vi "subvi2.vi"(10 "Numeric in":i32, 11 "Motor Step/Direction":u16) -> (3 "Numeric out":u32)   [LabVIEW 2018]
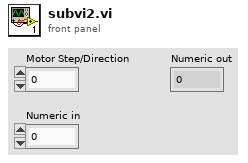
[diagram p1: front panel]
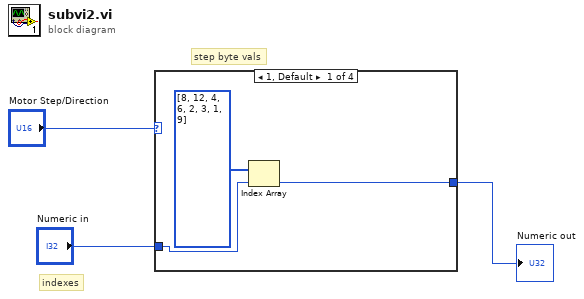
[diagram p0: block diagram]
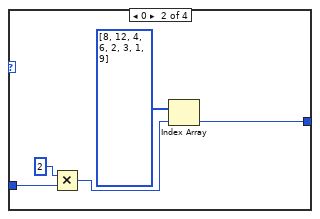
[diagram p2: hidden frame]
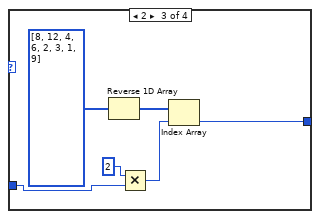
[diagram p3: hidden frame]
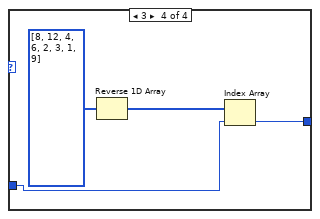
[diagram p4: hidden frame]
diagram:
  # "indexes"
  # "step byte vals"
  n1 = case shown="1, Default" "Motor Step/Direction" {
    tunnel: "Numeric in" -> [w5 w8 w12 w19]
    tunnel: [w4 w10 w13 w18] -> w2
    frame 1, Default {
      n2 = Index Array(array=u32[] [8, 12, 4, 6, 2, 3, 1, 9], index=w5) -> (element=w4:u32)
    }
    frame 0 {
      n3 = Multiply(x=2, y=w8) -> (x*y=w9:i32)
      n4 = Index Array(array=u32[] [8, 12, 4, 6, 2, 3, 1, 9], index=w9) -> (element=w10:u32)
    }
    frame 2 {
      n5 = Reverse 1D Array(array=u32[] [8, 12, 4, 6, 2, 3, 1, 9]) -> (reversed array=w14:u32[])
      n6 = Multiply(x=2, y=w12) -> (x*y=w17:i32)
      n7 = Index Array(array=w14, index=w17) -> (element=w13:u32)
    }
    frame 3 {
      n8 = Reverse 1D Array(array=u32[] [8, 12, 4, 6, 2, 3, 1, 9]) -> (reversed array=w20:u32[])
      n9 = Index Array "Index Array"(array=w20, index=w19) -> (element=w18:u32)
    }
  }
  "Numeric out" <- w2
